vi "Lift Loop.vi"(8 "error in (no error)":errorcluster) -> ()   [LabVIEW 2014]
doc: "This VI runs in parallel to other tasks. It can contain as many user-defined periodic loops as you need. These can carry out PID or other sorts of timed response."
uses:
  Robot Global Data.vi
  <vilib>/addons/control/pid/pid.llb/PID (DBL).vi
  <vilib>/addons/control/pid/NI_PID_pid.lvlib
panel:
  in  "Level 5":dbl=4000.0
  in  "Level 4":dbl=3980.0
  in  "Level 3":dbl=2983.0
  in  "Level 2":dbl=2150.0
  in  "Level 1":dbl=958.0
  in  "Level G":dbl
  in  "PID gains":T1={"proportional gain (Kc)"=0.002, "integral time (Ti, min)"=0.0, "derivative time (Td, min)"=0.0} {"derivative time (Td, min)" format="%.3f"; "integral time (Ti, min)" format="%.3f"; "proportional gain (Kc)" format="%.3f"}
  in  "output range":cluster{"output high":dbl, "output low":dbl}={"output high"=0.7, "output low"=-0.7} {"output low" format="%.2f"; "output high" format="%.2f"}
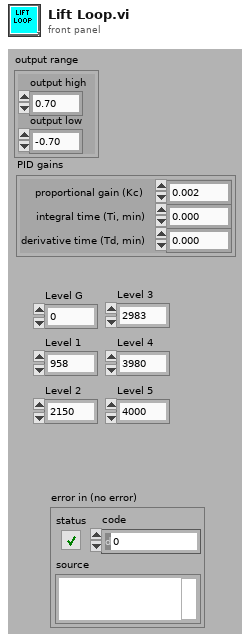
[diagram p1: front panel]
types:
  T1 = cluster{"proportional gain (Kc)":dbl, "integral time (Ti, min)":dbl, "derivative time (Td, min)":dbl}
  T2 = typedef "WPI_EncoderDevRef.ctl" = cluster{"DevStatus":errorcluster, "EncoderIndex":T3, "CounterIndex":T4, "DistancePerCount":dbl, "Decoding Type":T5}
  T3 = typedef "FPGA_EncoderIdx.ctl" = enum8{"Enc 0", "Enc 1", "Enc 2", "Enc 3", "Enc 4", "Enc 5", "Enc 6", "Enc 7", "Invalid"}
  T4 = typedef "FPGA_CounterCtrSystemIndex.ctl" = enum8{"Ctr 0", "Ctr 1", "Ctr 2", "Ctr 3", "Ctr 4", "Ctr 5", "Ctr 6", "Ctr 7", "Invalid"}
  T5 = typedef "WPI_EncoderType.ctl" = enum16{"1x", "2x", "4x"}
  T6 = typedef "WPI_MotorControlDeviceRef.ctl" = cluster{"DeviceStatus":errorcluster, "Type":T7, "PWM":cluster{"Controller":T8, "PWM Channel":T9, "DeadBand":T10}, "CAN":cluster{"Device Number":u8, "Control Mode":T11, "Semaphore":T12, "Max Vout":dbl, "TalonSRX Control Mode":T13}, "Invert":bool, "TransformRef":T14, "InvTransformRef":T14}
  T7 = typedef "WPI_MotorControlType.ctl" = enum16{"PWM", "CAN", "CANTalonSRX"}
  T8 = typedef "FPGA_TypedefDigitalModule.ctl" = enum16{"Controller 1"}
  T9 = typedef "FPGA_DIOPWMChannel.ctl" = enum8{"PWM 0", "PWM 1", "PWM 2", "PWM 3", "PWM 4", "PWM 5", "PWM 6", "PWM 7", "PWM 8", "PWM 9", "PWM MXP 0", "PWM MXP 1", "PWM MXP 2", "PWM MXP 3", "PWM MXP 4", "PWM MXP 5", "PWM MXP 6", "PWM MXP 7", "PWM MXP 8", "PWM MXP 9", "Invalid"}
  T10 = typedef "WPI_PWMDeadband.ctl" = cluster{"Name":string, "maxPositivePwm":i32, "minPositivePwm":i32, "centerPwm":i32, "maxNegativePwm":i32, "minNegativePwm":i32, "angularRange":u16}
  T11 = typedef "WPI_CANJaguar_ControlMode.ctl" = enum8{"Percent VBus", "Current", "Speed", "Position", "Voltage"}
  T12 = typedef "Semaphore RefNum" = refnum<k1>
  T13 = typedef "WPI_CANTalonSRX_APIControlMode.ctl" = enum8{"Percent VBus", "Speed", "Position", "Slave", "Unchanged / Invalid"}
  T14 = typedef "WPI_PWMTransform_ConPane.ctl" = refnum<vi>
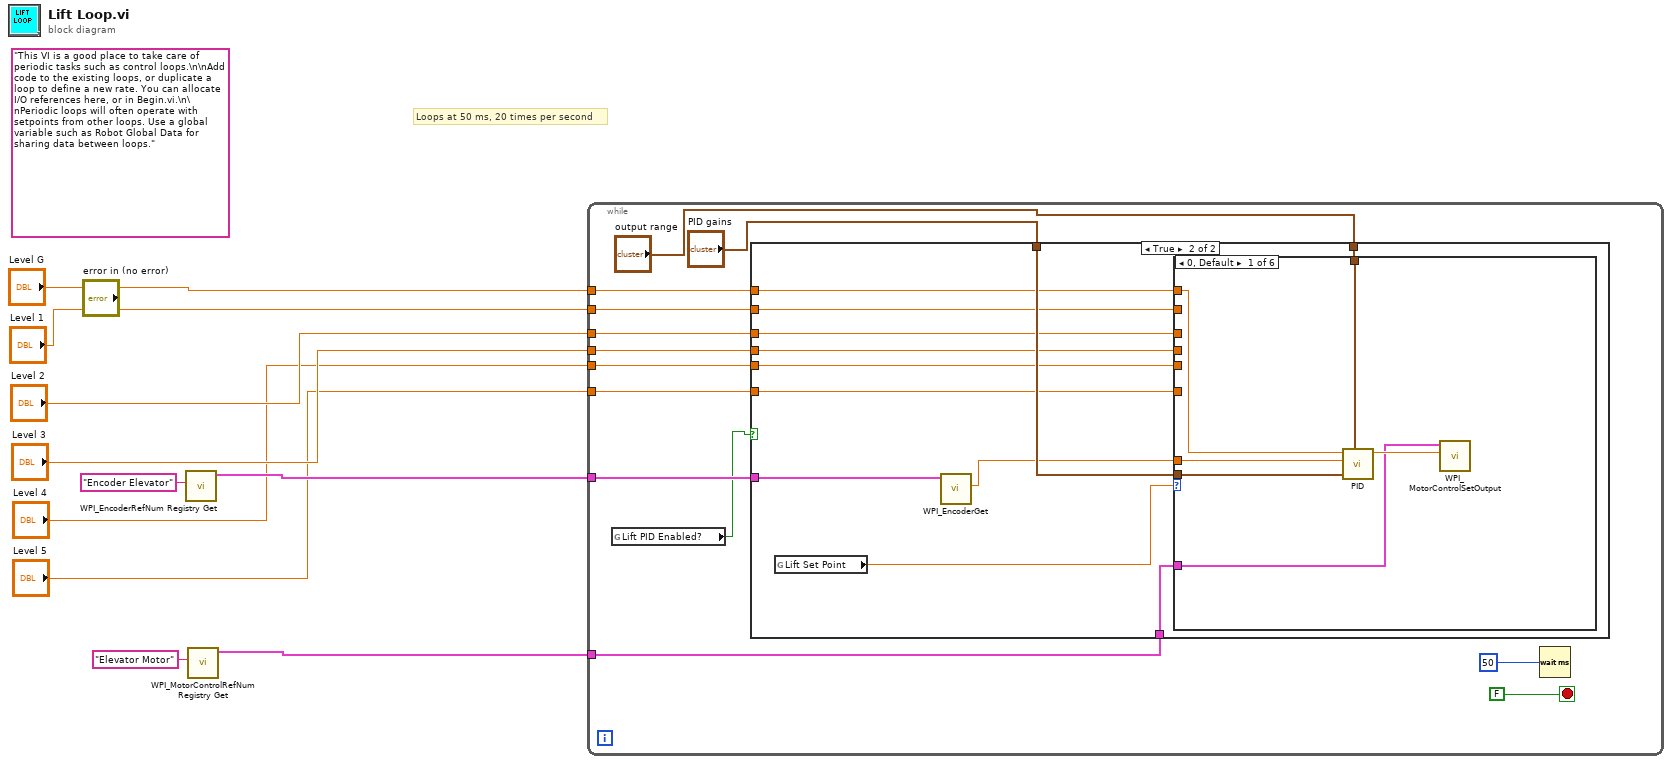
[diagram p0: block diagram]
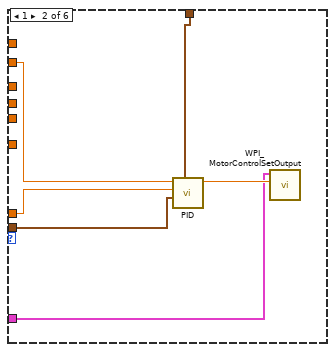
[diagram p3: hidden frame]
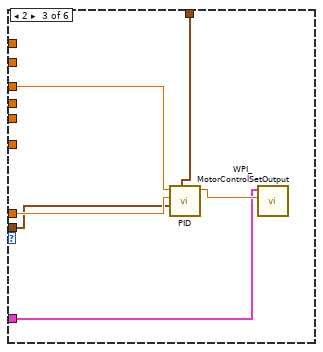
[diagram p4: hidden frame]
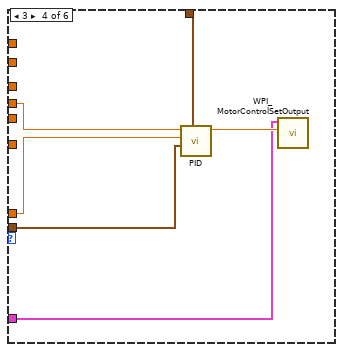
[diagram p5: hidden frame]
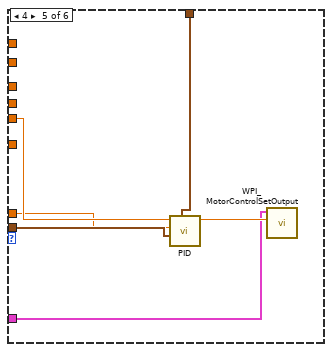
[diagram p6: hidden frame]
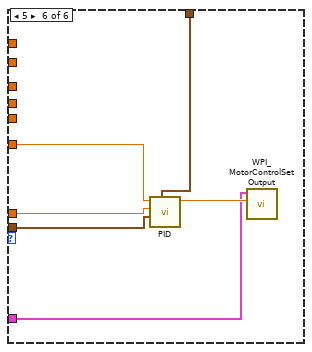
[diagram p7: hidden frame]
diagram:
  (unwired) "This VI is a good place to take care of periodic tasks such as control loops.\n\nAdd code to the existing loops, or duplicate a loop to define a new rate. You can allocate I/O references here, or in Begin.vi.\n\nPeriodic loops will often operate with setpoints from other loops. Use a global variable such as Robot Global Data for sharing data between loops."
  # "Loops at 50 ms, 20 times per second"
  n1 = call <vilib>:"WPI_EncoderRefNum Registry Get.vi"("refnum name"="Encoder Elevator") -> ("EncoderDevRef"=w9:T2)  [unwired: 9 in, 1 out]
  n2 = call <vilib>:"WPI_MotorControlRefNum Registry Get.vi"("refnum name"="Elevator Motor") -> ("MotorControlDevRef"=w1:T6)  [unwired: 9 in, 1 out]
  n3 = while {
    tunnel: w9 -> [w21]
    tunnel: "Level G" -> [w20]
    tunnel: "Level 1" -> [w19]
    tunnel: "Level 2" -> [w18]
    tunnel: "Level 3" -> [w17]
    tunnel: "Level 4" -> [w16]
    tunnel: "Level 5" -> [w15]
    tunnel: w1 -> [w14]
    stop <- FALSE stop-if-true
    n4 = global read "Robot Global Data.vi" "Lift PID Enabled?"() -> (w13:bool)
    n5 = case shown="True" w13 {
      tunnel: "output range" -> [_ w34]
      tunnel: "PID gains" -> [_ w33]
      tunnel: w21 -> [_ w32]
      tunnel: w20 -> [_ w30]
      tunnel: w19 -> [_ w29]
      tunnel: w18 -> [_ w28]
      tunnel: w17 -> [_ w27]
      tunnel: w16 -> [_ w26]
      tunnel: w15 -> [_ w25]
      tunnel: w14 -> [_ w24]
      frame False {
      }
      frame True {
        n6 = global read "Robot Global Data.vi" "Lift Set Point"() -> (w35:dbl)
        n7 = call <vilib>:"WPI_EncoderGet.vi"("EncoderDevRef"=w32) -> ("Distance"=w31:dbl)  [unwired: 5 in, 5 out]
        n8 = case shown="0, Default" w35 {
          tunnel: w34 -> [w41 w47 w50 w56 w65 w68]
          tunnel: w33 -> [w40 w46 w51 w57 w64 w69]
          tunnel: w31 -> [w39 w45 w52 w58 w62 w70]
          tunnel: w30 -> [w38 _ _ _ _ _]
          tunnel: w29 -> [_ w44 _ _ _ _]
          tunnel: w28 -> [_ _ w53 _ _ _]
          tunnel: w27 -> [_ _ _ w59 _ _]
          tunnel: w26 -> [_ _ _ _ w63 _]
          tunnel: w25 -> [_ _ _ _ _ w71]
          tunnel: w24 -> [w36 w42 w48 w54 w60 w66]
          frame 0, Default {
            n9 = call-poly <vilib>:"PID.vi"("output range"=w41, "PID gains"=w40, "process variable"=w39, "setpoint"=w38) -> ("output"=w37:dbl)  [unwired: 6 in, 1 out]
            n10 = call <vilib>:"WPI_MotorControlSetOutput.vi"("Output"=w37, "MotorControlDevRef"=w36) -> ()  [unwired: 7 in, 3 out]
          }
          frame 1 {
            n11 = call-poly <vilib>:"PID.vi"("output range"=w47, "PID gains"=w46, "process variable"=w45, "setpoint"=w44) -> ("output"=w43:dbl)  [unwired: 6 in, 1 out]
            n12 = call <vilib>:"WPI_MotorControlSetOutput.vi"("Output"=w43, "MotorControlDevRef"=w42) -> ()  [unwired: 7 in, 3 out]
          }
          frame 2 {
            n13 = call-poly <vilib>:"PID.vi"("output range"=w50, "PID gains"=w51, "process variable"=w52, "setpoint"=w53) -> ("output"=w49:dbl)  [unwired: 6 in, 1 out]
            n14 = call <vilib>:"WPI_MotorControlSetOutput.vi"("Output"=w49, "MotorControlDevRef"=w48) -> ()  [unwired: 7 in, 3 out]
          }
          frame 3 {
            n15 = call-poly <vilib>:"PID.vi"("output range"=w56, "PID gains"=w57, "process variable"=w58, "setpoint"=w59) -> ("output"=w55:dbl)  [unwired: 6 in, 1 out]
            n16 = call <vilib>:"WPI_MotorControlSetOutput.vi"("Output"=w55, "MotorControlDevRef"=w54) -> ()  [unwired: 7 in, 3 out]
          }
          frame 4 {
            n17 = call-poly <vilib>:"PID.vi"("output range"=w65, "PID gains"=w64, "process variable"=w62, "setpoint"=w63) -> ("output"=w61:dbl)  [unwired: 6 in, 1 out]
            n18 = call <vilib>:"WPI_MotorControlSetOutput.vi"("Output"=w61, "MotorControlDevRef"=w60) -> ()  [unwired: 7 in, 3 out]
          }
          frame 5 {
            n19 = call-poly <vilib>:"PID.vi"("output range"=w68, "PID gains"=w69, "process variable"=w70, "setpoint"=w71) -> ("output"=w67:dbl)  [unwired: 6 in, 1 out]
            n20 = call <vilib>:"WPI_MotorControlSetOutput.vi"("Output"=w67, "MotorControlDevRef"=w66) -> ()  [unwired: 7 in, 3 out]
          }
        }
      }
    }
    n21 = Wait (ms)(milliseconds to wait=u32 50) -> ()  [unwired: 1 out]
  }
